vi "6.4.vi"   [LabVIEW 2017]
uses:
  <vilib>/Utility/file.llb/Write Delimited Spreadsheet (DBL).vi
  <vilib>/measure/NI_MABase.lvlib
types:
  T1 = enum16{"open", "replace", "create", "open or create", "replace or create", "replace or create with confirmation"}
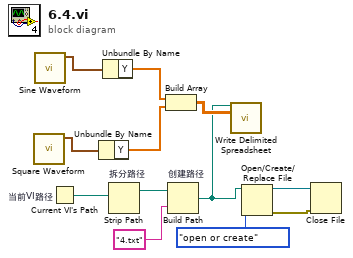
[diagram p0: block diagram]
diagram:
  n1 = call <vilib>:"Square Waveform.vi"() -> ("signal out"=w12:waveform(dbl))  [unwired: 10 in, 1 out]
  n2 = call <vilib>:"Sine Waveform.vi"() -> ("signal out"=w11:waveform(dbl))  [unwired: 10 in, 1 out]
  n3 = Current VI's Path "当前VI路径"() -> (path=w7:path)
  n4 = Unbundle By Name(w12) -> ("Y"=w9:dbl[])
  n5 = Unbundle By Name(w11) -> ("Y"=w10:dbl[])
  n6 = Strip Path "拆分路径"(path=w7) -> (stripped path=w6:path)  [unwired: 1 out]
  n7 = Build Array(w10, w9) -> (w8:dbl[][])
  n8 = Build Path "创建路径"(base path=w6, name or relative path="4.txt") -> (appended path=w5:path)
  n9 = call-poly <vilib>:"Write Delimited Spreadsheet.vi"("file path (dialog if empty)"=w5, "2D data"=w8) -> ()  [unwired: 12 in, 2 out]
  n10 = Open/Create/Replace File(file path (use dialog)=w5, operation (0:open)=T1."open or create" ("操作(0:open)")) -> (refnum out=w2:refnum<file>, error out=w1:errorcluster)  [unwired: 4 in, 1 out]
  n11 = Close File(refnum=w2, error in=w1) -> ()  [unwired: 2 out]
